vi "Update Log.vi"(8 "error in (no error)":errorcluster, 10 "Message":string, 11 "Test UI in":refnum<class "Test UI.lvclass">) -> (0 "error out":errorcluster, 3 "Test UI out":refnum<class "Test UI.lvclass">)   [LabVIEW 2024, in "Test UI.lvlib" / "Test UI.lvclass"]
uses:
  Test UI.lvclass
  Test UI.lvclass/Test UI.ctl
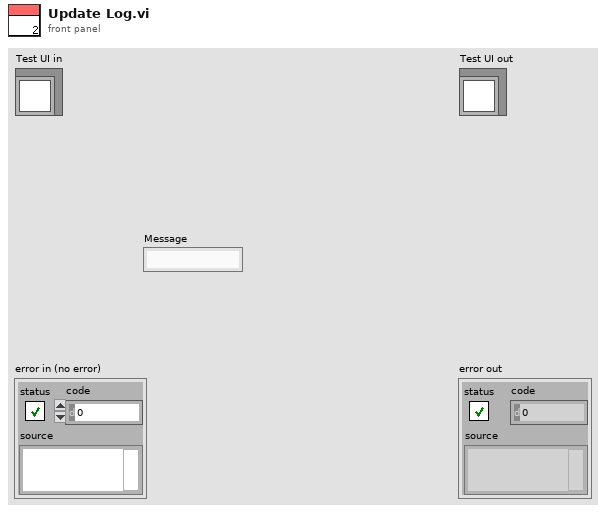
[diagram p1: front panel]
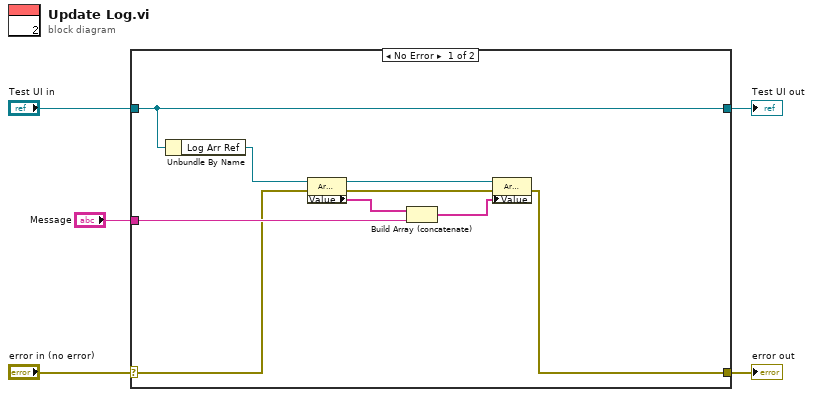
[diagram p0: block diagram]
diagram:
  n1 = case shown="No Error" "error in (no error)" {
    selector: "error in (no error)" -> [w7 w16]
    tunnel: [w6 w16] -> w4
    tunnel: [w14 w15] -> w2
    tunnel: "Test UI in" -> [w14 w15]
    tunnel: "Message" -> [w11 _]
    frame No Error {
      n2 = Unbundle By Name(w14) -> ("Log Arr Ref"=w13:refnum<vi>)
      n3 = property class="Arr (strict)"(reference=w13, error in=w7) -> (reference out=w10:refnum<vi>, error out=w9:errorcluster, "Value"=w12:string[])
      n4 = Build Array (concatenate)(w12, w11) -> (w8:string[])
      n5 = property class="Arr (strict)"(reference=w10, error in=w9, "Value"=w8) -> (error out=w6:errorcluster)  [unwired: 1 out]
    }
    frame Error {
    }
  }
  "error out" <- w4
  "Test UI out" <- w2
